vi "Magnetometer - Convert XY to NSEW Heading_SubVI.vi"(11 "Flux In (uT)":dbl[](array[numeric])) -> (2 "Heading Output (Str)":T1, 3 "Heading":dbl)   [LabVIEW 2021]
uses:
  Lab 5/Lab 5 Code/Heading_TDef.ctl
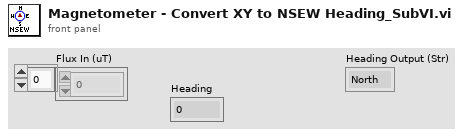
[diagram p1: front panel]
types:
  T1 = typedef "Heading_TDef.ctl" = enum16{"North ", "North East", "East", "Southeast", "South", "Southwest", "West", "Northwest"}
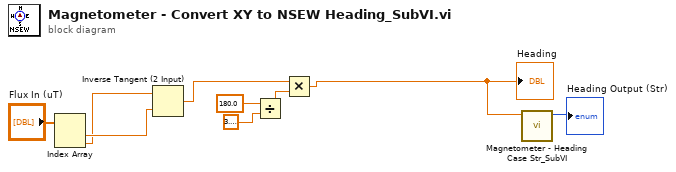
[diagram p0: block diagram]
diagram:
  n1 = Index Array(array="Flux In (uT)") -> (element #1=w2:dbl, element #2=w1:dbl)  [unwired: 2 in]
  n2 = Inverse Tangent (2 Input)(1:w2, 2:w1) -> (0:w9:dbl)
  n3 = Divide(x=180.0, y=3.141592653589793) -> (x/y=w8:dbl)
  n4 = Multiply(x=w9, y=w8) -> (x*y=w4:dbl)
  "Heading" <- w4
  n5 = call "Magnetometer - Heading Case Str_SubVI.vi"("Heading Input (deg)"=w4) -> ("Heading Output (Str)"=→"Heading Output (Str)":T1)  [unwired: 10 in]
